vi "set all Motor Ok.vi"(8 "error in (no error)":errorcluster, 11 "AISAS Motors":refnum<class "AISAS motor.lvclass">[](array[class])) -> (0 "error out":errorcluster, 3 "AISAS Motors out":refnum<class "AISAS motor.lvclass">[](array[class]))   [LabVIEW 2014, in "AISAS motor.lvclass"]
uses:
  AISAS motor.lvclass
  AISAS motor.lvclass/AISAS motor.ctl
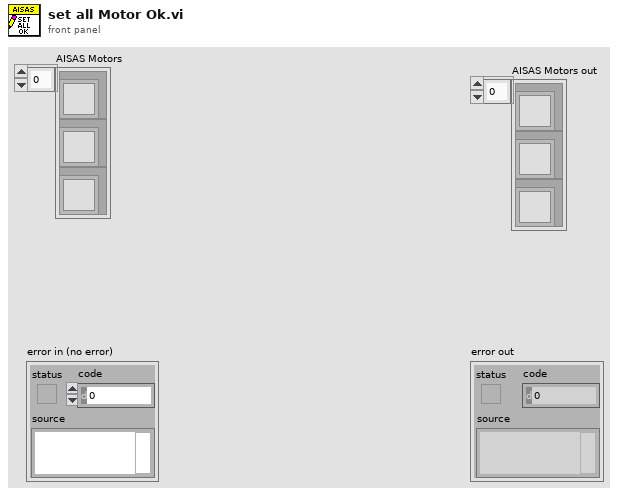
[diagram p1: front panel]
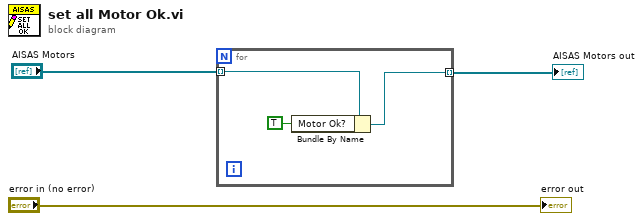
[diagram p0: block diagram]
diagram:
  n1 = for {
    tunnel: "AISAS Motors" -> [w6] mode=indexing
    tunnel: [w5] -> w1 mode=indexing
    n2 = Bundle By Name(cluster=w6, "Motor Ok?"=TRUE) -> (w5:refnum<class "AISAS motor.lvclass">)
  }
  "AISAS Motors out" <- w1
  "error out" <- "error in (no error)"
